vi "RSC_Init.vi"(8 "error in (no error)":errorcluster, 11 "Reward_SubCondition in":refnum<class "Reward_SubCondition.lvclass">) -> (0 "error out":errorcluster, 3 "Reward_SubCondition out":refnum<class "Reward_SubCondition.lvclass">)   [LabVIEW 2018, in "Tracker.lvlib" / "Reward_SubCondition.lvclass"]
uses:
  Reward_SubCondition.lvclass
  Reward_SubCondition.lvclass/Reward_SubCondition.ctl
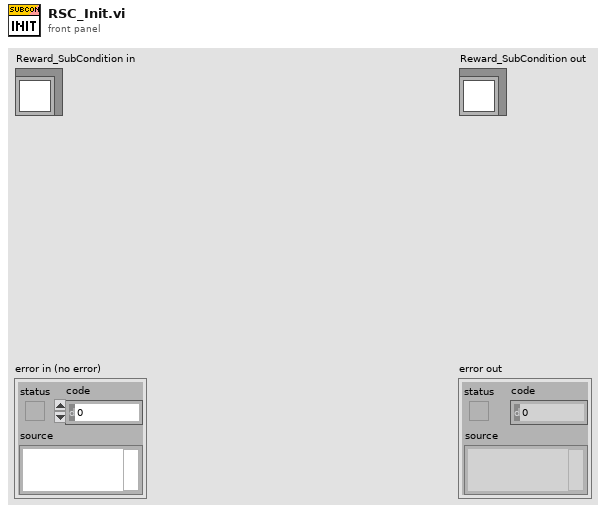
[diagram p1: front panel]
types:
  T1 = enum16{"Less", "Less or Equal", "Equal", "Greater or Equal", "Greater", "Not Equal"}
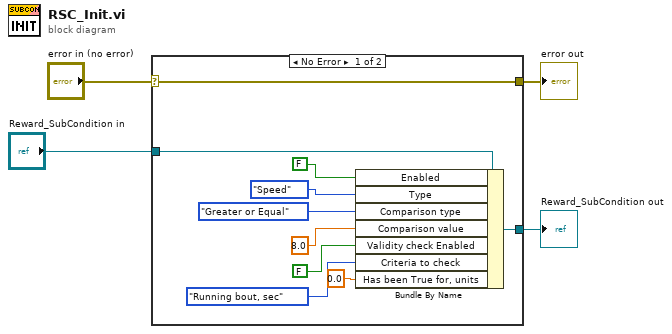
[diagram p0: block diagram]
diagram:
  n1 = case shown="No Error" "error in (no error)" {
    selector: "error in (no error)" -> [w14 w16]
    tunnel: [w14 w16] -> w3
    tunnel: [w12 w15] -> w1
    tunnel: "Reward_SubCondition in" -> [w13 w15]
    frame No Error {
      n2 = Bundle By Name(cluster=w13, "Enabled"=FALSE, "Type"=enum16{"Angle to wall", "Speed", "Zone"}."Speed", "Comparison type"=T1."Greater or Equal", "Comparison value"=8.0, "Validity check Enabled"=FALSE, "Criteria to check"=enum16{"Running bout, sec", "Running bout, m"}."Running bout, sec", "Has been True for, units"=0.0) -> (w12:refnum<class "Reward_SubCondition.lvclass">)
    }
    frame Error {
    }
  }
  "error out" <- w3
  "Reward_SubCondition out" <- w1
